vi "Base Ctrl Update Values.vi"(0 "Notifier Name In":string, 11 "Error In":errorcluster) -> (2 "Turret Filter":u32, 4 "Notifier Name Out":string, 6 "Obj Index":u32, 8 "Output Port":u32, 13 "Lamp Power":dbl, 14 "Lamp State":bool, 15 "Error Out":errorcluster)   [LabVIEW 2020]
uses:
  Device Library/Microscopes/Polymorphic Microscope Messenger/Get Turret Filter.vi
  Device Library/Microscopes/Polymorphic Microscope Messenger/Get Obj Index.vi
  Device Library/Microscopes/Polymorphic Microscope Messenger/Get Output Port.vi
  Device Library/Microscopes/Polymorphic Microscope Messenger/Get Lamp Power.vi
  Device Library/Microscopes/Polymorphic Microscope Messenger/Get Lamp State.vi
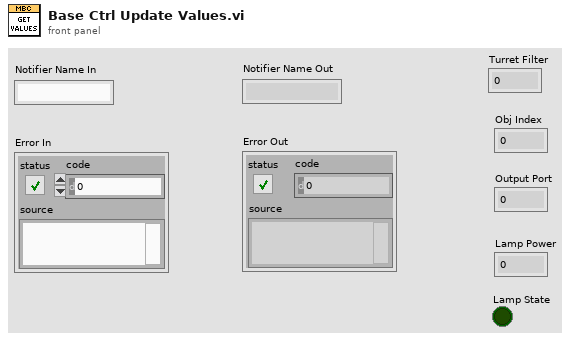
[diagram p1: front panel]
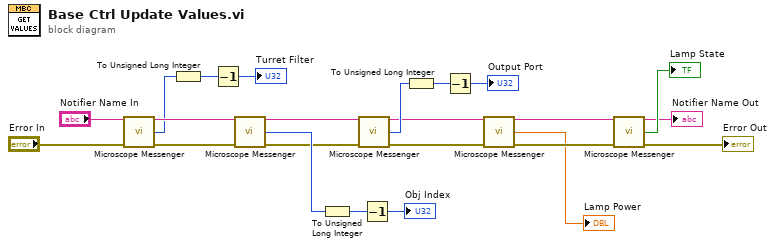
[diagram p0: block diagram]
diagram:
  n1 = call-poly "Microscope Messenger.vi"("Notifier Name In"="Notifier Name In", "Error In"="Error In") -> ("Notifier Name Out"=w19:string, "Turret Filter Index"=w17:u8, "Error Out"=w16:errorcluster)  [unwired: 11 in]
  n2 = To Unsigned Long Integer(number=w17) -> (unsigned 32bit integer=w18:u32)
  n3 = Decrement(x=w18) -> (x-1=→"Turret Filter":u32)
  n4 = call-poly "Microscope Messenger.vi"("Notifier Name In"=w19, "Error In"=w16) -> ("Notifier Name Out"=w2:string, "Objective Index"=w23:u8, "Error Out"=w1:errorcluster)  [unwired: 11 in]
  n5 = To Unsigned Long Integer(number=w23) -> (unsigned 32bit integer=w20:u32)
  n6 = call-poly "Microscope Messenger.vi"("Notifier Name In"=w2, "Error In"=w1) -> ("Notifier Name Out"=w9:string, "Output Port"=w22:u8, "Error Out"=w8:errorcluster)  [unwired: 11 in]
  n7 = Decrement(x=w20) -> (x-1=→"Obj Index":u32)
  n8 = To Unsigned Long Integer(number=w22) -> (unsigned 32bit integer=w21:u32)
  n9 = Decrement(x=w21) -> (x-1=→"Output Port":u32)
  n10 = call-poly "Microscope Messenger.vi"("Notifier Name In"=w9, "Error In"=w8) -> ("Notifier Name Out"=w14:string, "Lamp Power (%)"=→"Lamp Power":dbl, "Error Out"=w15:errorcluster)  [unwired: 11 in]
  n11 = call-poly "Microscope Messenger.vi"("Notifier Name In"=w14, "Error In"=w15) -> ("Notifier Name Out"=→"Notifier Name Out":string, "Lamp State"=→"Lamp State":bool, "Error Out"=→"Error Out":errorcluster)  [unwired: 11 in]
